vi "Sequencer Do.vi"(8 "error in (no error)":errorcluster, 10 "Sequencer in":refnum<class "Sequencer.lvclass">, 11 "Batch End Msg":refnum<class "Batch End Msg.lvclass">) -> (0 "error out":errorcluster, 2 "Sequencer out":refnum<class "Sequencer.lvclass">)   [LabVIEW 2020, in "Sequencer.lvlib" / "Batch End Msg.lvclass"]
doc: "The action the Sequencer Msg performs in the Sequencers Recieve Message method.\n\nThis implementation does nothing."
uses:
  Batch End Msg.lvclass
  Sequencer/Sequencer.lvclass
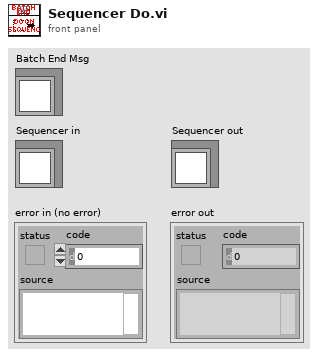
[diagram p1: front panel]
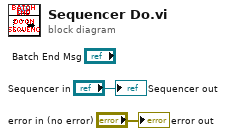
[diagram p0: block diagram]
diagram:
  "error out" <- "error in (no error)"
  "Sequencer out" <- "Sequencer in"
